vi "Move Part.vi"(8 "Place":bool caption="Pick", 9 "Offset":cluster{"x":dbl, "y":dbl, "a":dbl}={"x"=50.0, "y"=900.0, "a"=900.0}, 10 "Location":string="Large Gear", 11 "Part Name":string="Large Gear") -> (0 "error out":errorcluster)   [LabVIEW 2013]
uses:
  ROS/Code/SubVIs/BaxterSide.ctl
  <vilib>/Analysis/Matrix/Datatypes/RealMatrix.ctl
  <vilib>/Analysis/Matrix/Numeric/Multiply/Multiply - RM,RM.vi
  ROS/Code/Console/Servers/ServerSubs/(nist) Arm Globals.vi
  Arm Globals.vi
  Move/Move Matrix.vi
  <vilib>/Analysis/Matrix/NI_Matrix.lvlib
panel:
  in  "side":T1=enum."right"
  # "Y"
  # "X"
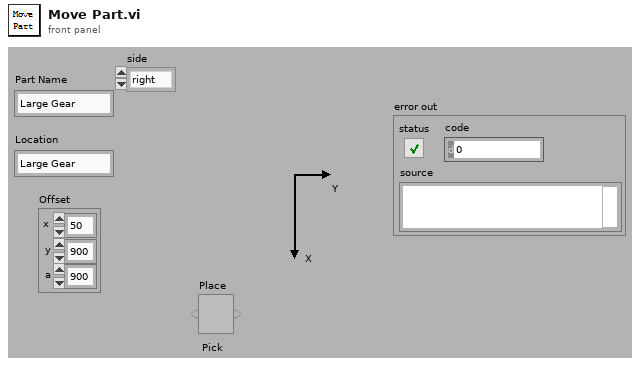
[diagram p1: front panel]
types:
  T1 = typedef "BaxterSide.ctl" = enum16{"left", "right"}
  T2 = typedef "NI_Matrix.lvlib/RealMatrix.ctl" = dbl[][]
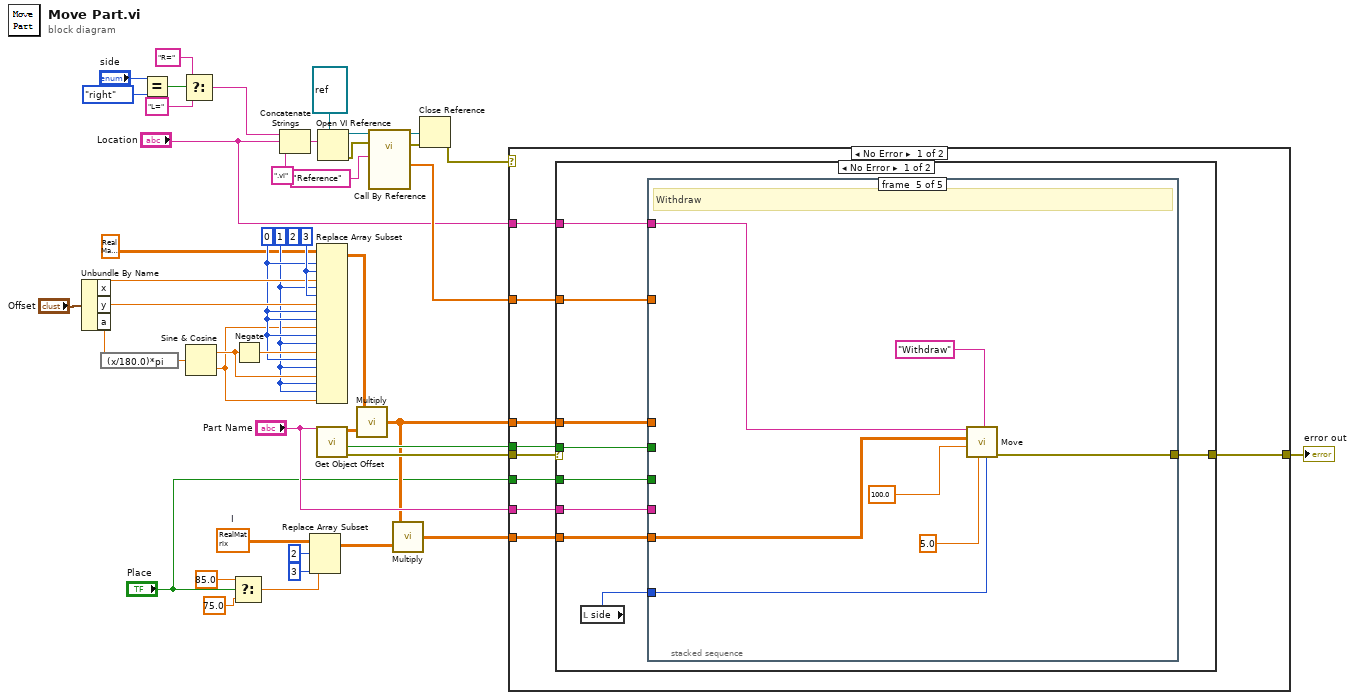
[diagram p0: block diagram]
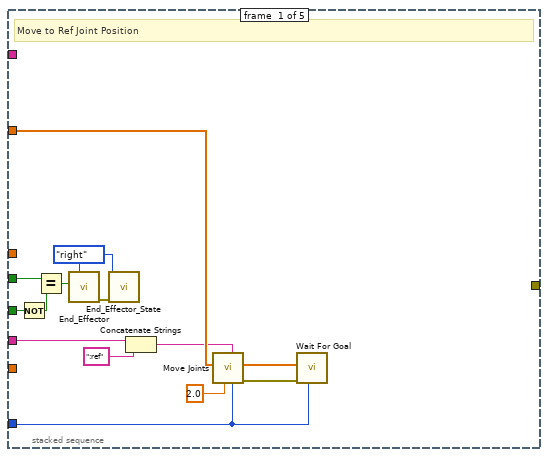
[diagram p2: hidden frame]
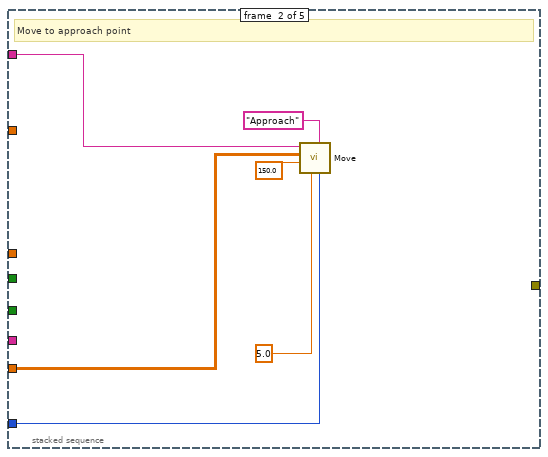
[diagram p3: hidden frame]
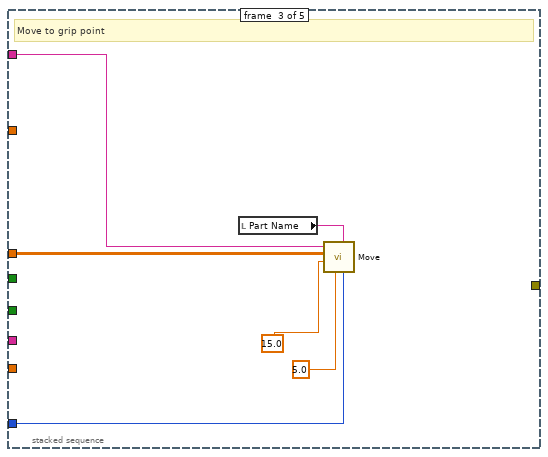
[diagram p4: hidden frame]
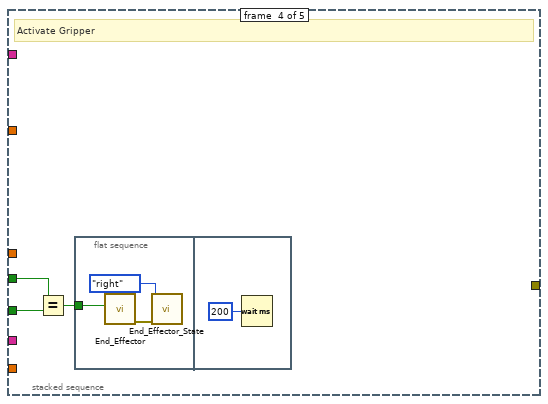
[diagram p5: hidden frame]
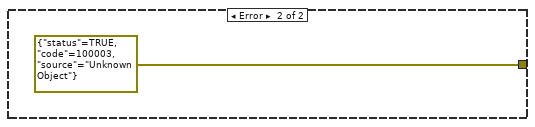
[diagram p6: hidden frame]
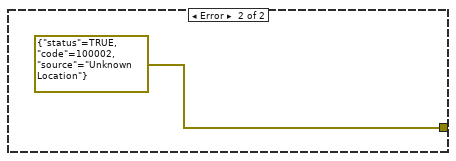
[diagram p7: hidden frame]
diagram:
  w30 = T2 [[1.0, 0.0, 0.0, 0.0], [0.0, 1.0, 0.0, 0.0], [0.0, 0.0, 1.0, 0.0], [0.0, 0.0, 0.0, 1.0]]  # I
  (unwired) 2 ("disabled index (row)")
  w36 = 1 ("disabled index (row)")
  w44 = 3 ("disabled index (col)")
  w38 = 0 ("disabled index (row)")
  n1 = Unbundle By Name("Offset") -> ("x"=w42:dbl, "y"=w41:dbl, "a"=w40:dbl)
  n2 = expression code="(x/180.0)*pi" ("degrees to radians")(w40) -> (w43:dbl)
  n3 = Equal?(x="side", y=BaxterSide."right" ("Side")) -> (x = y?=w16:bool)
  n4 = Select(t="R=", s=w16, f="L=") -> (s? t:f=w13:string)
  n5 = Sine & Cosine(0:w43) -> (1:w37:dbl, 2:w35:dbl)
  n6 = Select(t=85.0, s="Place", f=75.0 ("new element/submatrix")) -> (s? t:f=w3:dbl)
  n7 = Negate(x=w37) -> (-x=w39:dbl)
  n8 = Concatenate Strings(w13, "Location", ".vi" ("string")) -> (w25:string)
  n9 = Replace Array Subset(array=w30, new element=w3, index (row)=2 ("disabled index (row)"), index (col)=3 ("disabled index (col)")) -> (w27:T2)
  n10 = Replace Array Subset(array=T2 [[1.0, 0.0, 0.0, 0.0], [0.0, 1.0, 0.0, 0.0], [0.0, 0.0, 1.0, 0.0], [0.0, 0.0, 0.0, 1.0]] ("T"), new element #1=w42, index (row) #1=w38, index (col) #1=w44, new element #2=w41, index (row) #2=w36, index (col) #2=w44, new element #3=w35, index (row) #3=w38, index (col) #3=w38, new element #4=w39, index (row) #4=w38, index (col) #4=w36, new element #5=w37, index (row) #5=w38, index (col) #5=w36, new element #6=w35, index (row) #6=w36, index (col) #6=w36) -> (w32:T2)
  n11 = call "Get Object Offset.vi"("Label"="Part Name") -> ("error out"=w10:errorcluster, "GraspClose"=w8:bool, "T"=w31:T2)  [unwired: 7 in, 1 out]
  n12 = Open VI Reference(type specifier VI Refnum (for type only)=refnum<vi> refnum, vi path=w25) -> (vi reference=w23:refnum<vi>, error out=w20:errorcluster)  [unwired: 4 in]
  n13 = call-poly <vilib>:"Multiply.vi"("Real Matrix B"=w31, "Real Matrix A"=w32) -> ("A * B"=w5:T2)
  n14 = call-by-ref "?"(reference=w23, error in=w20, "Command"="Reference") -> (reference out=w21:refnum<vi>, error out=w19:errorcluster, "Joints"=w12:dbl[])  [unwired: 8 in, 2 out]
  n15 = call-poly <vilib>:"Multiply.vi"("Real Matrix B"=w27, "Real Matrix A"=w5) -> ("A * B"=w7:T2)
  n16 = Close Reference(reference=w21, error in (no error)=w19) -> (error out=w11:errorcluster)
  n17 = case shown="No Error" w11 {
    tunnel: [w54 errorcluster {"status"=TRUE, "code"=100002, "source"="Unknown Location"} ("error out")] -> w45
    tunnel: w12 -> [w52 _]
    tunnel: w10 -> [w53 _]
    tunnel: "Part Name" -> [w51 _]
    tunnel: w8 -> [w50 _]
    tunnel: w7 -> [w49 _]
    tunnel: "Location" -> [w48 _]
    tunnel: w5 -> [w47 _]
    tunnel: "Place" -> [w46 _]
    frame No Error {
      n18 = case shown="No Error" w53 {
        tunnel: [w63 errorcluster {"status"=TRUE, "code"=100003, "source"="Unknown Object"} ("error out")] -> w54
        tunnel: w50 -> [w62 _]
        tunnel: w52 -> [w60 _]
        tunnel: w51 -> [w59 _]
        tunnel: w49 -> [w58 _]
        tunnel: w48 -> [w57 _]
        tunnel: w47 -> [w56 _]
        tunnel: w46 -> [w55 _]
        frame No Error {
          n19 = local read "side"() -> (w61:T1)
          n20 = stacked-sequence {
            tunnel: w61 -> [w65 w78 w84 _ w99]
            tunnel: [_ _ _ _ w97] -> w63
            tunnel: w55 -> [w74 _ _ w92 _]
            tunnel: w59 -> [w70 _ _ _ _]
            tunnel: w62 -> [w72 _ _ w90 _]
            tunnel: w60 -> [w69 _ _ _ _]
            tunnel: w58 -> [_ w81 _ _ w101]
            tunnel: w57 -> [_ w80 w86 _ w100]
            tunnel: w56 -> [_ _ w87 _ _]
            frame #0 {
              w76 = BaxterSide."right" ("Side")
              # "Move to Ref Joint Position"
              n21 = Not(x=w74) -> (.not. x?=w73:bool)
              n22 = Equal?(x=w72, y=w73) -> (x = y?=w71:bool)
              n23 = call "End_Effector.vi"("Close"=w71, "Side"=w76) -> ("error out"=w75:errorcluster)  [unwired: 6 in]
              n24 = call "End_Effector_State.vi"("error in"=w75, "Side"=w76) -> ()  [unwired: 4 in, 3 out]
              n25 = Concatenate Strings(w70, ":ref" ("string")) -> (w67:string)
              n26 = call "Move Joints.vi"("Side"=w65, "Label"=w67, "Wait (s)"=2.0, "Goal"=w69) -> ("error out"=w66:errorcluster, "Goal"=w64:dbl[])  [unwired: 6 in]
              n27 = call "Wait For Goal.vi"("Side"=w65, "error in"=w66, "Goal"=w64) -> ()  [unwired: 7 in, 2 out]
            }
            frame #1 {
              # "Move to approach point"
              n28 = call-poly "Move.vi"("Side"=w78, "Label"="Approach", "Wait Time"=5.0 ("milliseconds to wait"), "Speed (mm/s)"=150.0, "Offset"=w81, "Location"=w80) -> ()  [unwired: 5 in, 1 out]
            }
            frame #2 {
              # "Move to grip point"
              n29 = local read "Part Name"() -> (w85:string)
              n30 = call-poly "Move.vi"("Side"=w84, "Label"=w85, "Wait Time"=5.0 ("milliseconds to wait"), "Speed (mm/s)"=15.0, "Offset"=w87, "Location"=w86) -> ()  [unwired: 5 in, 1 out]
            }
            frame #3 {
              # "Activate Gripper"
              n31 = Equal?(x=w90, y=w92) -> (x = y?=w91:bool)
              n32 = flat-sequence {
                tunnel: w91 -> [w93]
                frame #0 {
                  w95 = BaxterSide."right" ("Side")
                  n33 = call "End_Effector.vi"("Close"=w93, "Side"=w95) -> ("error out"=w94:errorcluster)  [unwired: 6 in]
                  n34 = call "End_Effector_State.vi"("error in"=w94, "Side"=w95) -> ()  [unwired: 4 in, 3 out]
                }
                frame #1 {
                  n35 = Wait (ms)(milliseconds to wait=u32 200) -> ()  [unwired: 1 out]
                }
              }
            }
            frame #4 {
              # "Withdraw"
              n36 = call-poly "Move.vi"("Side"=w99, "Label"="Withdraw", "Wait Time"=5.0 ("milliseconds to wait"), "Speed (mm/s)"=100.0, "Offset"=w101, "Location"=w100) -> ("error out"=w97:errorcluster)  [unwired: 5 in]
            }
          }
        }
        frame Error {
        }
      }
    }
    frame Error {
    }
  }
  "error out" <- w45
